vi "Create.vi"(7 "Direction":T1, 8 "error in (no error)":errorcluster, 9 "Custom Config Data":u8[](array[numeric]), 10 "Name":string, 11 "CIFTag in":refnum<class "CIF_CIPC_Chn_Double.lvclass">) -> (0 "error out":errorcluster, 3 "CIFTag out":refnum<class "CIF_CIPC_Chn_Double.lvclass">)   [LabVIEW 2021, in "CIF_CIPC_Chn_Double.lvclass"]
uses:
  CIF_CIPC_Chn_Double.lvclass
  D:/dev/Packages/CIF_Channels_Core/src/CIFChannels/CIFChannels.lvclass
  D:/dev/Packages/CIF_Channels_Core/src/CIPC_Channels/CIF_CIPC_Chan/CIF_CIPC_Chn.lvclass
  CIFChannels/Typedef/Direction.ctl
  CIFChannels/Typedef/Disconnect Behavior.ctl
  ChannelCommon/typedef/Channel Pattern.ctl
  CIFChannels/CIFChannels.lvclass/CIFChannels.ctl
  CIFChannels/Typedef/Channel State.ctl
  CIF_CIPC_Chan/Typedef/Buffer Configuration Data.ctl
  CIF_CIPC_Chan/CIF_CIPC_Chn.lvclass/CIF_CIPC_Chn.ctl
  CIF_CIPC_Chn_Double.lvclass/CIF_CIPC_Chn_Double.ctl
  df6797b5-3f3a-463f-a676-d85c8ce06da0.vi
  3e71386b-e635-4616-ad06-93410a9d2207.vi
  CIF_CIPC_Chan/Accessors/Write CIPC Channel.vi
  CIF_CIPC_Chan/Accessors/Write Buffer Configuration.vi
  CIFChannels/Accessors/Write Channel State.vi
  CIFChannels/Accessors/Write Pattern.vi
  CIFChannels/SubVIs/Get Type from Class.vi
  ChannelCommon/Utilities/Unflatten FIFO Config.vi
  CIFChannels/Utilities/Apply Flags.vi
  CIFChannels/Accessors/Write Type.vi
  CIFChannels/Accessors/Write Channel Class.vi
  CIFChannels/Accessors/Write Direction.vi
  CIFChannels/Accessors/Write Tag Disconnect Behavior.vi
  CIFChannels/Accessors/Write Name.vi
  CIFChannels/Accessors/Write Custom Config Data.vi
  df6797b5-3f3a-463f-a676-d85c8ce06da0.vi/49b3dd2d-4579-4089-b72e-3f0875c862f2.vi
  <vilib>/CIF Foundation/CIF CIPC/SubVIs/Check Error.vi
  <vilib>/CIF Foundation/CIF CIPC/SubVIs/Get dll Path.vi
  <vilib>/CIF Foundation/CIF CIPC/SubVIs/Get Element Write Position.vi
  <vilib>/CIF Foundation/CIF CIPC/SubVIs/Notify Of New Write.vi
  <vilib>/CIF Foundation/CIF Utilities/DataTypes/Flatten Unflatten/Unflatten U64.vi
  ChannelCommon/Utilities/Expand FIFO Flags.vi
  <vilib>/Utility/LVClass/Get LV Class Name.vi
  <vilib>/CIF Foundation/CIF CIPC/SubVIs/Get Element Description Variant.vi
  <vilib>/Utility/error.llb/Trim Whitespace.vi
  <vilib>/string/Create NI GUID.vi
  <vilib>/Utility/error.llb/Error Cluster From Error Code.vi
  <vilib>/CIF Foundation/CIF CIPC/SubVIs/Get Element Info Variant.vi
  CIFChannels/CIFChannels.lvclass
  <vilib>/CIF Foundation/CIF CIPC/CIF_NI_CIPC.lvlib
  CIF_CIPC_Chan/CIF_CIPC_Chn.lvclass
  ChannelCommon/ChannelCommon.lvlib
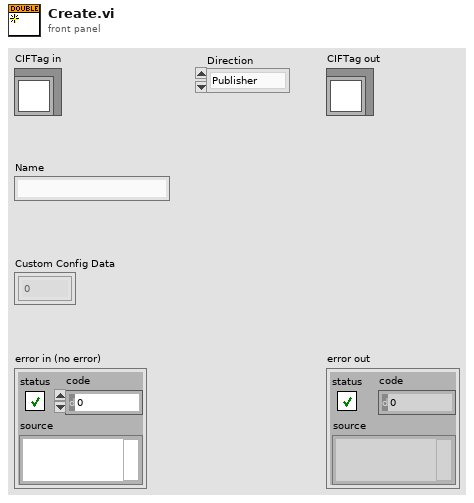
[diagram p1: front panel]
types:
  T1 = typedef "CIFChannels.lvclass/Direction.ctl" = enum16{"Publisher", "Subscriber"}
  T2 = typedef "ChannelCommon.lvlib/Channel Pattern.ctl" = enum16{"Unknown", "Tag", "FIFO", "MultiFIFO"}
  T3 = typedef "CIFChannels.lvclass/Disconnect Behavior.ctl" = enum16{"Default value", "Last value", "Error with default"}
  T4 = typedef "CIF_CIPC_Chn.lvclass/Buffer Configuration Data.ctl" = cluster{"Total Size":u32, "Read Size":u32, "Read Offset":u32, "Encoder Data":string}
  T5 = typedef "CIFChannels.lvclass/Channel State.ctl" = enum16{"Creating", "Disconnected", "Connecting", "Connected", "Destroyed"}
  T6 = typedef "CIF_NI_CIPC.lvlib/Encoder Info.ctl" = cluster{"Name":string, "Version":i32, "Data":string}
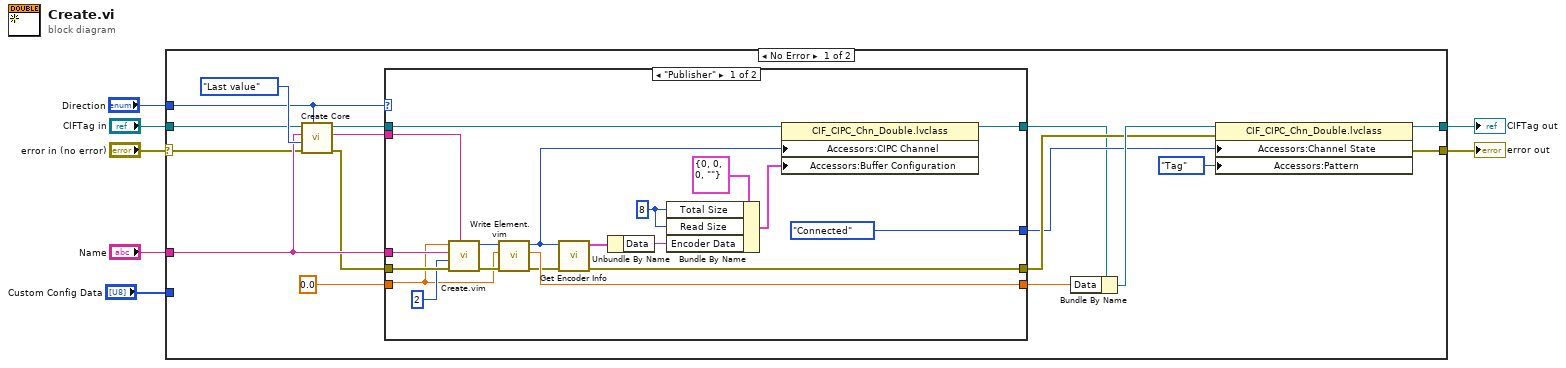
[diagram p0: block diagram]
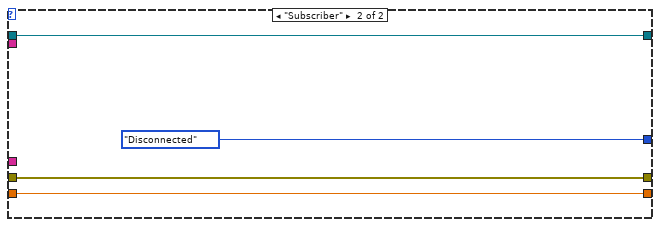
[diagram p2: hidden frame]
diagram:
  n1 = case shown="No Error" "error in (no error)" {
    selector: "error in (no error)" -> [w14 w49]
    tunnel: [w23 w49] -> w1
    tunnel: [w18 w48] -> w5
    tunnel: "CIFTag in" -> [w13 w48]
    tunnel: "Name" -> [w22 _]
    tunnel: "Direction" -> [w17 _]
    tunnel: "Custom Config Data" -> [_ _]
    frame No Error {
      n2 = call "Create Core.vi"("Direction"=w17, "error in (no error)"=w14, "Disconnect Behavior"=Disconnect_Behavior."Last value", "Name"=w22, "CIFChannels in"=w13) -> ("error out"=w12:errorcluster, "Channel Type"=w10:string, "CIFChannels out"=w9:refnum<class "CIF_CIPC_Chn_Double.lvclass">)  [unwired: 2 in, 2 out]
      n3 = case shown="\"Publisher\"" w17 {
        tunnel: w22 -> [w39 _]
        tunnel: w12 -> [w40 w45]
        tunnel: 0.0 ("Default Value") -> [w36 w46]
        tunnel: [w35 w46] -> w20
        tunnel: [w26 w45] -> w19
        tunnel: [Channel_State."Connected" ("Channel State") Channel_State."Disconnected" ("Channel State")] -> w16
        tunnel: w10 -> [w37 _]
        tunnel: w9 -> [w34 w44]
        tunnel: [w25 w44] -> w8
        frame "Publisher" {
          w27 = u32 8 ("Total Size")
          n4 = call "Create.vim"("Description"=w37, "error in (no error)"=w40, "Buffer Size N (2^N)"=u8 2, "Name in"=w39, "Data Type"=w36) -> ("error out"=w41:errorcluster, "CIPC Reference"=w42:u64)  [unwired: 3 in, 2 out]
          n5 = call "Write Element.vim"("error in (no error)"=w41, "Data in"=w36, "CIPC Reference in"=w42) -> ("error out"=w33:errorcluster, "Data out"=w35:dbl, "CIPC Reference out"=w32:u64)  [unwired: 5 in, 1 out]
          n6 = call <vilib>:"Get Encoder Info.vi"("error in (no error)"=w33, "CIPC Reference"=w32) -> ("error out"=w26:errorcluster, "Encoder Info"=w31:T6)  [unwired: 8 in]
          n7 = Unbundle By Name(w31) -> ("Data"=w30:string)
          n8 = Bundle By Name(cluster=T4 {"Total Size"=0, "Read Size"=0, "Read Offset"=0, "Encoder Data"=""} ("Buffer Configuration"), "Total Size"=w27, "Read Size"=w27, "Encoder Data"=w30) -> (w29:T4)
          n9 = property class="CIF_CIPC_Chn_Double.lvclass"(reference=w34, "Accessors:CIPC Channel"=w32, "Accessors:Buffer Configuration"=w29) -> (reference out=w25:refnum<class "CIF_CIPC_Chn_Double.lvclass">)  [unwired: 1 in, 1 out]
        }
        frame "Subscriber" {
        }
      }
      n10 = Bundle By Name(cluster=w8, "Data"=w20) -> (w21:refnum<class "CIF_CIPC_Chn_Double.lvclass">)
      n11 = property class="CIF_CIPC_Chn_Double.lvclass"(reference=w21, error in=w19, "Accessors:Channel State"=w16, "Accessors:Pattern"=Channel_Pattern."Tag" ("Pattern")) -> (reference out=w18:refnum<class "CIF_CIPC_Chn_Double.lvclass">, error out=w23:errorcluster)
    }
    frame Error {
    }
  }
  "error out" <- w1
  "CIFTag out" <- w5
